vi "Disabled.vi"(7 "Robot Mode":T2, 10 "Match Info":T1={"Autonomous Elapsed Seconds"=0.0, "TeleOp Elapsed Seconds"=0.0, "Disabled Elapsed Seconds"=0.0, "Visited Autonomous"=FALSE, "Visited TeleOp"=FALSE, "Visited Disabled"=FALSE, "Autonomous Settings"={"Autonomous Style"=enum."Independent", "VI Refnum"=refnum}}, 11 "Call Context":T3) -> ()   [LabVIEW 2019]
doc: "This VI is called each time a disabled packet is received from the DS. It is often used to prepare for the next robot mode, to calibrate sensors, etc."
uses:
  <vilib>/Rock Robotics/WPI/DriverStation/WPI_DriverStationDerivedRobotMode.ctl
  <vilib>/Rock Robotics/WPI/DriverStation/WPI_DriverStationRobotMode2.ctl
  <vilib>/Rock Robotics/WPI/DriverStation/WPI_DriverStationMatch Info.ctl
  InfiniteRechargeSrc/Global_Var-RefNum/JoystickControls.vi
  InfiniteRechargeSrc/TypeDefs/JoystickControl.ctl
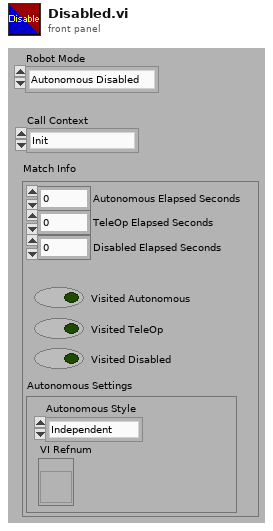
[diagram p1: front panel]
types:
  T1 = typedef "WPI_DriverStationMatch Info.ctl" = cluster{"Autonomous Elapsed Seconds":dbl, "TeleOp Elapsed Seconds":dbl, "Disabled Elapsed Seconds":dbl, "Visited Autonomous":bool, "Visited TeleOp":bool, "Visited Disabled":bool, "Autonomous Settings":cluster{"Autonomous Style":enum16{"Iterative", "Independent"}, "VI Refnum":refnum<vi>}}
  T2 = typedef "WPI_DriverStationRobotMode2.ctl" = enum16{"Autonomous Disabled", "Autonomous Enabled", "Teleop Disabled", "Teleop Enabled", "Disconnected", "Finish", "Test Disabled", "Test Enabled", "Emergency Stopped"}
  T3 = typedef "WPI_DriverStationDerivedRobotMode.ctl" = enum16{"Init", "Execute", "Stop"}
  T4 = typedef "JoystickControl.ctl" = cluster{"A":bool, "B":bool, "X":bool, "Y":bool, "LB":bool, "Shoot":bool, "LJ":bool, "RJ":bool, "Back":bool, "Start":bool, "Top":bool, "Right":bool, "Bottom":bool, "Left":bool, "Eject":dbl, "Intake":dbl, "LX":dbl, "Drive Y":dbl, "Drive X":dbl, "RY":dbl, "Down":bool, "Index":bool, "Aggitate":bool, "Up":bool, "Find Target":bool, "Spin up":bool, "LJ 2":bool, "RJ 2":bool, "Back 2":bool, "Start 2":bool, "Elevate":bool, "Right 2":bool, "Retract":bool, "Left 2":bool, "Control Rotate":dbl, "RT 2":dbl, "H L/R":dbl, "H U/D":dbl, "RX 2":dbl, "RY 2":dbl}
  T5 = typedef "JoystickRefNums.ctl" = cluster{"Joystick0":T6, "Joystick1":T6}
  T6 = typedef "WPI_JoystickDevRef.ctl" = cluster{"Device":T7}
  T7 = typedef "WPI_JoystickDeviceEnum.ctl" = enum16{"USB 0", "USB 1", "USB 2", "USB 3", "USB 4", "USB 5"}
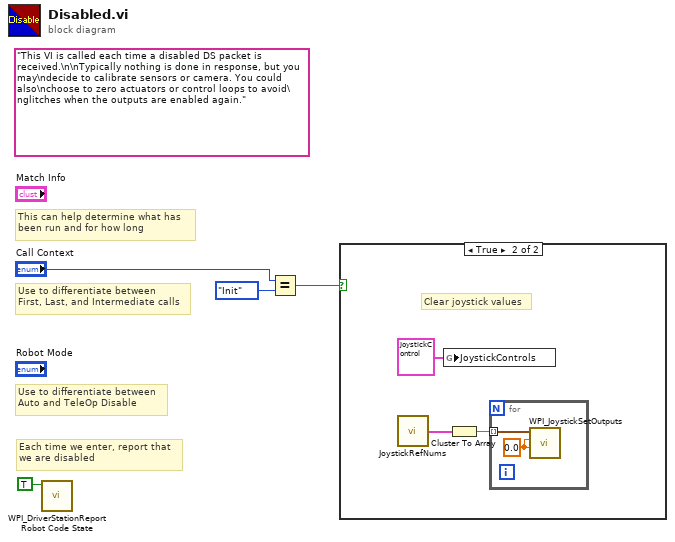
[diagram p0: block diagram]
diagram:
  (unwired) "This VI is called each time a disabled DS packet is received.\n\nTypically nothing is done in response, but you may\ndecide to calibrate sensors or camera. You could also\nchoose to zero actuators or control loops to avoid\nglitches when the outputs are enabled again."
  # "Each time we enter, report that\nwe are disabled"
  # "Use to differentiate between\nFirst, Last, and Intermediate calls"
  # "This can help determine what has\nbeen run and for how long"
  # "Use to differentiate between\nAuto and TeleOp Disable"
  n1 = call <vilib>:"WPI_DriverStationReport Robot Code State.vi"("Disabled"=TRUE ("Autonomous")) -> ()  [unwired: 10 in, 1 out]
  n2 = Equal?(x="Call Context", y=WPI_DriverStationDerivedRobotMode."Init") -> (x = y?=w1:bool)
  n3 = case shown="True" w1 {
    frame False {
    }
    frame True {
      # "Clear joystick values"
      n4 = call "JoystickRefNums.vi"() -> ("JoystickRefNums"=w6:T5)  [unwired: 1 in]
      n5 = global write "JoystickControls.vi" "JoystickControls"(T4 {"A"=FALSE, "B"=FALSE, "X"=FALSE, "Y"=FALSE, "LB"=FALSE, "Shoot"=FALSE, "LJ"=FALSE, "RJ"=FALSE, "Back"=FALSE, "Start"=FALSE, "Top"=FALSE, "Right"=FALSE, "Bottom"=FALSE, "Left"=FALSE, "Eject"=0.0, "Intake"=0.0, "LX"=0.0, "Drive Y"=0.0, "Drive X"=0.0, "RY"=0.0, "Down"=FALSE, "Index"=FALSE, "Aggitate"=FALSE, "Up"=FALSE, "Find Target"=FALSE, "Spin up"=FALSE, "LJ 2"=FALSE, "RJ 2"=FALSE, "Back 2"=FALSE, "Start 2"=FALSE, "Elevate"=FALSE, "Right 2"=FALSE, "Retract"=FALSE, "Left 2"=FALSE, "Control Rotate"=0.0, "RT 2"=0.0, "H L/R"=0.0, "H U/D"=0.0, "RX 2"=0.0, "RY 2"=0.0} ("JoystickControls")) -> ()
      n6 = Cluster To Array(cluster=w6) -> (array=w5:T6[])
      n7 = for {
        tunnel: w5 -> [w9] mode=indexing
        w8 = sgl 0.0 ("Right Rumble")
        n8 = call <vilib>:"WPI_JoystickSetOutputs.vi"("Right Rumble"=w8, "Left Rumble"=w8, "JoystickDevRef"=w9) -> ()  [unwired: 7 in, 2 out]
      }
    }
  }
